vi "Auto_Routine_BlueRightTwoPieceTRAJ.vi"   [LabVIEW 2023]
uses:
  Trajectory/TrajectoryGlobals.vi
  <vilib>/Rock Robotics/WPI/ThirdParty/JAS_Junk/TrajLib/Trajectory_Library.lvlib
types:
  T1 = typedef "Trajectory_Library.lvlib/TRAJECTORY.ctl" = cluster{"TotalTImeSecs":dbl, "States":T2[]}
  T2 = typedef "Trajectory_Library.lvlib/TRAJ_STATE.ctl" = cluster{"TimeSeconds":dbl, "Velocity":dbl, "Acceleration":dbl, "POSE":T3, "Curvature":dbl}
  T3 = typedef "Trajectory_Library.lvlib/POSE2D.ctl" = cluster{"TRANSLATION":T4, "ROTATION":T5}
  T4 = typedef "Trajectory_Library.lvlib/TRANSLATION2D.ctl" = cluster{"X":dbl, "Y":dbl}
  T5 = typedef "Trajectory_Library.lvlib/ROTATION2D.ctl" = cluster{"VALUE":dbl, "COS":dbl, "SIN":dbl}
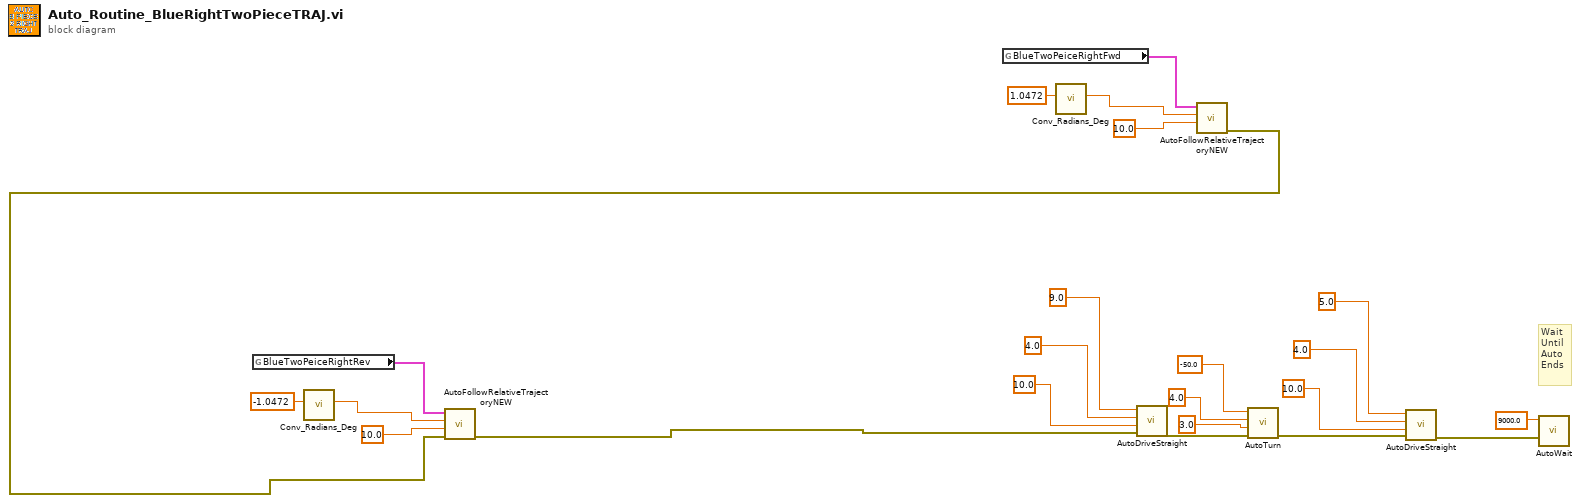
[diagram p0: block diagram]
diagram:
  # "Wait\nUntil\nAuto \nEnds"
  n1 = global read "TrajectoryGlobals.vi" "BlueTwoPeiceRightRev"() -> (w18:T1)
  n2 = call <vilib>:"Conv_Radians_Deg.vi"("Radians"=-1.0472) -> ("Degrees"=w16:dbl)  [unwired: 10 in]
  n3 = global read "TrajectoryGlobals.vi" "BlueTwoPeiceRightFwd"() -> (w23:T1)
  n4 = call <vilib>:"Conv_Radians_Deg.vi"("Radians"=1.0472) -> ("Degrees"=w21:dbl)  [unwired: 10 in]
  n5 = call "AutoFollowRelativeTrajectoryNEW.vi"("TimeOut (s)"=10.0, "End Orientation"=w21, "Trajectory"=w23) -> ("error out"=w2:errorcluster)  [unwired: 8 in]
  n6 = call "AutoFollowRelativeTrajectoryNEW.vi"("error in (no error)"=w2, "TimeOut (s)"=10.0, "End Orientation"=w16, "Trajectory"=w18) -> ("error out"=w1:errorcluster)  [unwired: 7 in]
  n7 = call "AutoDriveStraight.vi"("error in (no error)"=w1, "TimeOut (s)"=10.0, "MaxSpeed (ft/s)"=4.0, "Dist (ft)"=9.0) -> ("error out"=w6:errorcluster)  [unwired: 7 in]
  n8 = call "AutoTurn.vi"("error in (no error)"=w6, "TimeOut (s)"=3.0, "MaxSpeed (ft/s)"=4.0, "degrees"=-50.0) -> ("error out"=w8:errorcluster)  [unwired: 7 in]
  n9 = call "AutoDriveStraight.vi"("error in (no error)"=w8, "TimeOut (s)"=10.0, "MaxSpeed (ft/s)"=4.0, "Dist (ft)"=5.0) -> ("error out"=w7:errorcluster)  [unwired: 7 in]
  n10 = call "AutoWait.vi"("error in (no error)"=w7, "TimeOut (s)"=9000.0) -> ()  [unwired: 9 in, 1 out]
